vi "select frequency (subVI).vi"(9 "upper limit":dbl=26000.0, 10 "lower limit":dbl=24000.0, 11 "Original Signal":dbl[](array[numeric])) -> (1 "frequency 2":dbl, 2 "frequency 1":dbl, 3 "Portion":dbl[](array[numeric]))   [LabVIEW 2012]
uses:
  <vilib>/Analysis/NI_AALPro.lvlib
panel:
  in  "Portion Duration":i32=4000
  out "Original Spectrum 2":waveform(dbl)(graph)
  out "Signal 2":dbl[](graph)
  out "Original Spectrum":waveform(dbl)(graph)
  out "Signal 1":dbl[](graph)
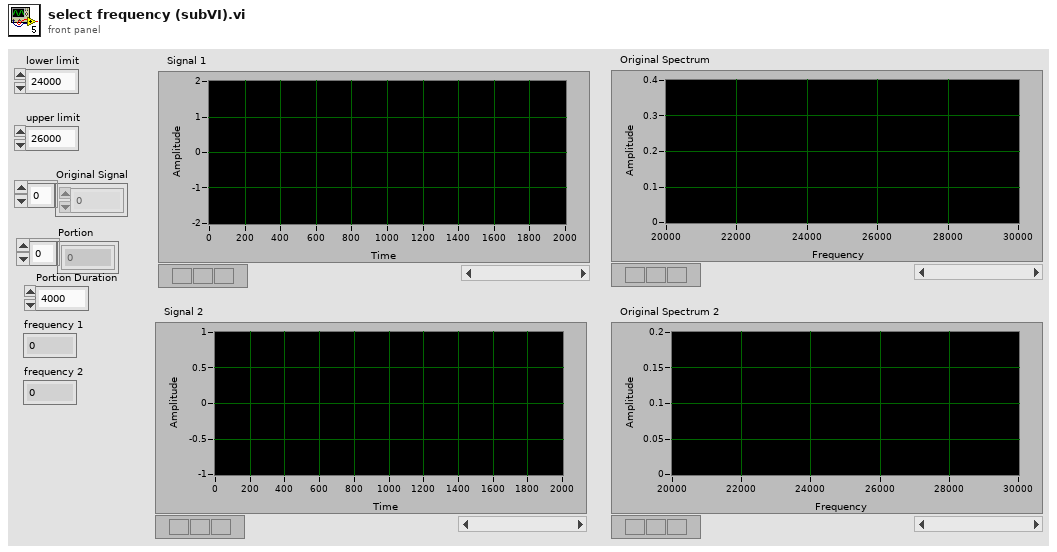
[diagram p1: front panel]
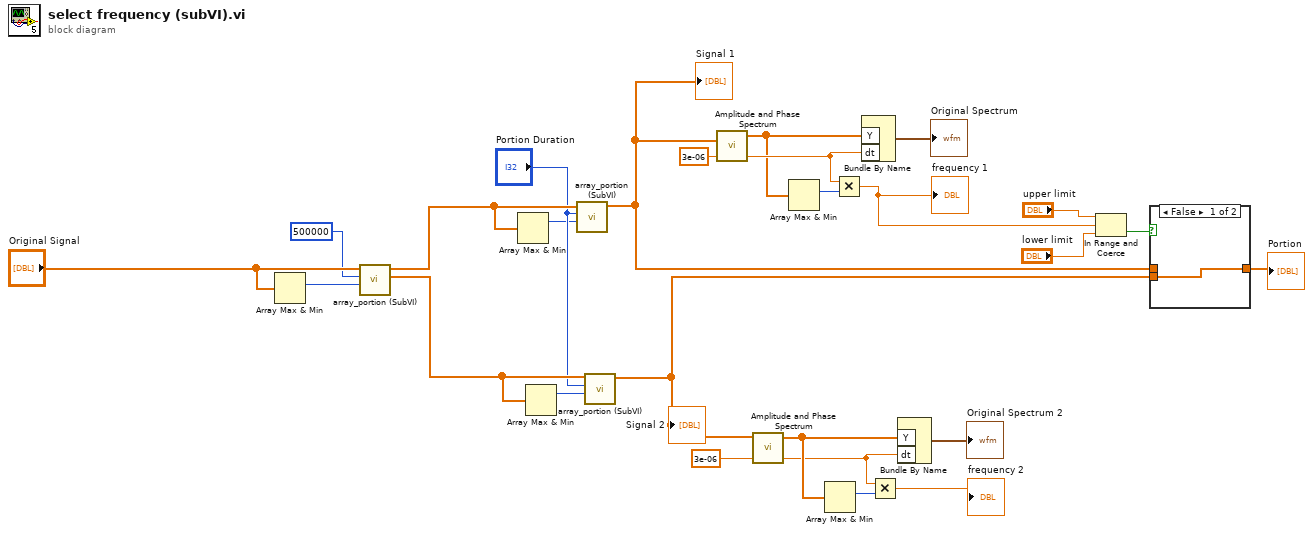
[diagram p0: block diagram]
diagram:
  n1 = Array Max & Min(array="Original Signal") -> (max index (indices)=w1:i32)  [unwired: 3 out]
  n2 = call "array_portion (SubVI).vi"("Starting Point"=w1, "Portion Duration"=500000, "Input Array"="Original Signal") -> ("Remain"=w23:dbl[], "Portion"=w22:dbl[])  [unwired: 7 in]
  n3 = Array Max & Min(array=w22) -> (max index (indices)=w6:i32)  [unwired: 3 out]
  n4 = Array Max & Min(array=w23) -> (max index (indices)=w14:i32)  [unwired: 3 out]
  n5 = call "array_portion (SubVI).vi"("Starting Point"=w6, "Portion Duration"="Portion Duration", "Input Array"=w22) -> ("Portion"=w25:dbl[])  [unwired: 7 in, 1 out]
  "Signal 1" <- w25
  n6 = call "array_portion (SubVI).vi"("Starting Point"=w14, "Portion Duration"="Portion Duration", "Input Array"=w23) -> ("Portion"=w26:dbl[])  [unwired: 7 in, 1 out]
  "Signal 2" <- w26
  n7 = call <vilib>:"Amplitude and Phase Spectrum.vi"("dt"=3e-06, "Signal (V)"=w25) -> ("df"=w8:dbl, "Amp Spectrum Mag (Vrms)"=w7:dbl[])  [unwired: 1 in, 1 out]
  n8 = call <vilib>:"Amplitude and Phase Spectrum.vi"("dt"=3e-06, "Signal (V)"=w26) -> ("df"=w12:dbl, "Amp Spectrum Mag (Vrms)"=w13:dbl[])  [unwired: 1 in, 1 out]
  n9 = Array Max & Min(array=w7) -> (max index (indices)=w9:i32)  [unwired: 3 out]
  n10 = Array Max & Min(array=w13) -> (max index (indices)=w11:i32)  [unwired: 3 out]
  n11 = Multiply(x=w8, y=w9) -> (x*y=w20:dbl)
  "frequency 1" <- w20
  n12 = Bundle By Name("Y"=w7, "dt"=w8) -> (→"Original Spectrum":waveform(dbl))  [unwired: 1 in]
  n13 = Multiply(x=w12, y=w11) -> (x*y=→"frequency 2":dbl)
  n14 = Bundle By Name("Y"=w13, "dt"=w12) -> (→"Original Spectrum 2":waveform(dbl))  [unwired: 1 in]
  n15 = In Range and Coerce(upper limit="upper limit", x=w20, lower limit="lower limit") -> (In Range?=w21:bool)  [unwired: 1 out]
  n16 = case shown="False" w21 {
    tunnel: w25 -> [_ w28]
    tunnel: w26 -> [w27 _]
    tunnel: [w27 w28] -> w24
    frame False {
    }
    frame True {
    }
  }
  "Portion" <- w24
